vi "Autonomous Independent.vi"() -> ()   [LabVIEW 2015]
doc: "This VI is called when autonomous begins, and will automatically be terminated when autonomous ends. You can carry out timed or sensor driven robot movement independently without needing to return to the caller."
uses:
  Global Variables/refnum names.vi
panel:
  out "ACTUAL Loop Time":u32
  # "Be sure to right-click and choose Data Operations>>Make Current Value default if you want to save the array values with the VI"
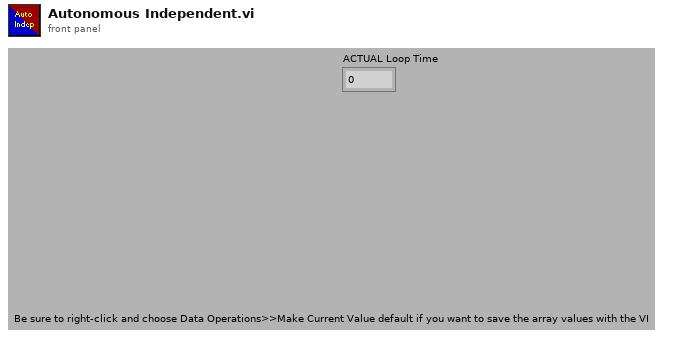
[diagram p1: front panel]
types:
  T1 = typedef "WPI_MotorControlDeviceRef.ctl" = cluster{"DeviceStatus":errorcluster, "Type":T2, "PWM":cluster{"PWM Channel":T3, "DeadBand":T4}, "CAN":cluster{"Device Number":u8, "Control Mode":T5, "Semaphore":T6, "Max Vout":dbl, "TalonSRX Control Mode":T7}, "Invert":bool}
  T2 = typedef "WPI_MotorControlType.ctl" = enum16{"PWM", "CAN", "CANTalonSRX"}
  T3 = typedef "FPGA_DIOPWMChannel.ctl" = enum8{"PWM 0", "PWM 1", "PWM 2", "PWM 3", "PWM 4", "PWM 5", "PWM 6", "PWM 7", "PWM 8", "PWM 9", "PWM MXP 0", "PWM MXP 1", "PWM MXP 2", "PWM MXP 3", "PWM MXP 4", "PWM MXP 5", "PWM MXP 6", "PWM MXP 7", "PWM MXP 8", "PWM MXP 9", "Invalid"}
  T4 = typedef "WPI_PWMDeadband.ctl" = cluster{"Name":string, "maxPositivePwm":i32, "minPositivePwm":i32, "centerPwm":i32, "maxNegativePwm":i32, "minNegativePwm":i32, "angularRange":u16}
  T5 = typedef "WPI_CANJaguar_ControlMode.ctl" = enum8{"Percent VBus", "Current", "Speed", "Position", "Voltage"}
  T6 = typedef "Semaphore RefNum" = refnum<k1>
  T7 = typedef "WPI_CANTalonSRX_APIControlMode.ctl" = enum8{"Percent VBus", "Speed", "Position", "Slave", "Unchanged / Invalid", "Voltage Compensation", "Current", "Motion Profile"}
  T8 = typedef "Autonomous Play Definition.ctl" = cluster{"Play Name":string, "Command List":cluster{"Param 1":dbl, "Param 2":dbl, "Autonomous Command Name":T9, "Concurrent":bool, "Param 3":dbl, "Param 4":string}[], "Play Description":string}
  T9 = typedef "Autonomous Command Names.ctl" = enum16{"No Op", "Drive Time", "Run Motion Profile", "Turn to Heading", "Turn To Target", "Cross Defense", "Fire", "Wait", "Reset Gyro", "Grabber Setpoints", "Manual Grabber", "Roller", "Autorange Command", "Reposition", "Drive Distance"}
  T10 = typedef "Robot Commands 2016.ctl" = cluster{"Robot Forward-Back":dbl, "Robot Twist":dbl, "Fire":bool, "Lift/Drive Shift":bool, "Raise Lifter":bool, "Raise Grabber":bool, "Lower Grabber":bool, "Roller":T11, "Robot Climb Both Sides":dbl, "Grabber to Middle Position":bool, "Grabber to Top Position":bool, "Grabber to Bottom Position":bool, "Robot Climb Left Side":dbl, "Robot Climb Right Side":dbl, "Speed Control Left Side":dbl, "Speed Control Right Side":dbl, "Lower Lifter":bool, "Defense Mode":bool, "Deploy Lifter":bool, "Auto Targetting":bool, "Do the Jiggle":bool}
  T11 = typedef "Roller State.ctl" = enum16{"DONT MOVE", "Intake", "Outtake"}
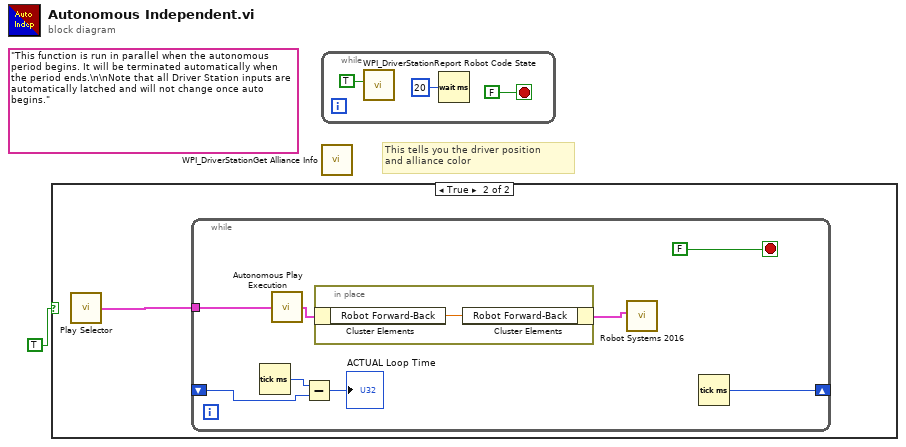
[diagram p0: block diagram]
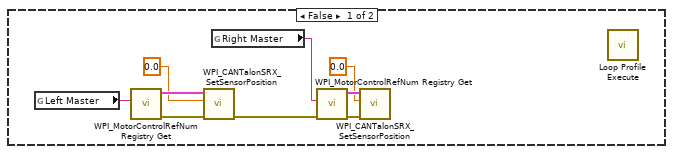
[diagram p2: hidden frame]
diagram:
  (unwired) "This function is run in parallel when the autonomous period begins. It will be terminated automatically when the period ends.\n\nNote that all Driver Station inputs are automatically latched and will not change once auto begins."
  # "This tells you the driver position\nand alliance color"
  n1 = case shown="True" TRUE {
    frame False {
      n2 = global read "refnum names.vi" "Left Master"() -> (w2:string)
      n3 = call <vilib>:"WPI_MotorControlRefNum Registry Get.vi"("refnum name"=w2) -> ("error out"=w10:errorcluster, "MotorControlDevRef"=w9:T1)  [unwired: 9 in]
      n4 = call <vilib>:"WPI_CANTalonSRX_SetSensorPosition.vi"("error in (no error)"=w10, "New Sensor Position"=0.0, "CAN Talon SRX Ref"=w9) -> ("error out"=w7:errorcluster)  [unwired: 7 in, 1 out]
      n5 = global read "refnum names.vi" "Right Master"() -> (w3:string)
      n6 = call <vilib>:"WPI_MotorControlRefNum Registry Get.vi"("error in (no error)"=w7, "refnum name"=w3) -> ("error out"=w5:errorcluster, "MotorControlDevRef"=w6:T1)  [unwired: 8 in]
      n7 = call <vilib>:"WPI_CANTalonSRX_SetSensorPosition.vi"("error in (no error)"=w5, "New Sensor Position"=0.0, "CAN Talon SRX Ref"=w6) -> ()  [unwired: 7 in, 2 out]
      n8 = call "Loop Profile Execute.vi"() -> ()  [unwired: 12 in]
    }
    frame True {
      n9 = call "Play Selector.vi"() -> ("Output Play"=w11:T8)  [unwired: 1 in]
      n10 = while {
        tunnel: w11 -> [w17]
        shift-right: [w15] -> _
        shift-left: _ -> [w14]
        stop <- FALSE stop-if-true
        n11 = Tick Count (ms)() -> (millisecond timer value=w13:u32)
        n12 = call "Autonomous Play Execution.vi"("Input Play"=w17) -> ("Robot System Functions"=w18:T10)
        n13 = Subtract(x=w13, y=w14) -> (x-y=→"ACTUAL Loop Time":u32)
        n14 = in-place {
          n15 = in-place-cluster #1(w18) -> ("Robot Forward-Back"=w20:dbl)
          n16 = in-place-cluster #1("Robot Forward-Back"=w20) -> (w16:T10)
        }
        n17 = call "Robot Systems 2016.vi"("Robot Commands"=w16) -> ()  [unwired: 11 in]
        n18 = Tick Count (ms)() -> (millisecond timer value=w15:u32)
      }
    }
  }
  n19 = while {
    stop <- FALSE stop-if-true
    n20 = call <vilib>:"WPI_DriverStationReport Robot Code State.vi"("Autonomous"=TRUE) -> ()  [unwired: 10 in, 1 out]
    n21 = Wait (ms)(milliseconds to wait=u32 20) -> ()  [unwired: 1 out]
  }
  n22 = call <vilib>:"WPI_DriverStationGet Alliance Info.vi"() -> ()  [unwired: 12 out]
